vi "Top Level FPGA_w8LED.vi"() -> ()   [LabVIEW 2012]
uses:
  <vilib>/Platform/TimedLoop/XDataNode/timing_clust.ctl
  <vilib>/Platform/TimedLoop/XDataNode/nitl_modes.ctl
  <vilib>/Platform/TimedLoop/XDataNode/wakeup.ctl
  <vilib>/rvi/DataTransferAndStorage/Container/Common/niFpgaContainerMetaDataKey.ctl
  <vilib>/rvi/DataTransferAndStorage/Container/Common/niFpgaContainerState.ctl
  <vilib>/rvi/DataTransferAndStorage/Container/Common/niFpgaDataTypeControl.ctl
  <vilib>/rvi/DataTransferAndStorage/Container/Common/niFpgaContainerImplementationControl.ctl
  <vilib>/rvi/DataTransferAndStorage/Container/Common/niFpgaContainerArbitrationOptionsControl.ctl
  <vilib>/rvi/DataTransferAndStorage/Container/Common/niFpgaTransferTypeControl.ctl
  <vilib>/rvi/DataTransferAndStorage/Container/Common/niFpgaContainerInitializationParameters.ctl
  <vilib>/rvi/Memory/Memory_Types/niFpgaMemoryInterfaceConfiguration.ctl
  <vilib>/rvi/FIFO/Fifo_Types/niFpgaFifoControlLogicControl.ctl
  <vilib>/rvi/eio/common/nirviEmuTemplateMethod_errors.vi
  <vilib>/rvi/FIFO/Fifo_Resource/nirvififoEmulationSetSize.vi
  <vilib>/rvi/DataTransferAndStorage/Container/Common/niFpgaContainerGetUniqueNameForEmu.vi
  <vilib>/rvi/Emulation/niFpgaSctlEmulationRegisterWithScheduler.vi
  <vilib>/rvi/Emulation/niFpgaSctlEmulationScheduler.vi
  <vilib>/rvi/DataTransferAndStorage/Container/Common/niFpgaContainerSetEmuInfo.vi
  <vilib>/rvi/eio/common/nirviEmuReportErrorAndStop.vi
  <vilib>/rvi/Emulation/niFpgaSctlEmulationFifoFullMgr.vi
  <vilib>/rvi/errors/niFpgaSetErrorForExecOnDevCompSimple.vi
  <vilib>/rvi/Memory/Memory_Emulation/niFpgaMemoryEmulationCacheClearOnFirstRun.vi
  <vilib>/rvi/Memory/Memory_Emulation/nirvimemoryEmulationManagerCache_MakeExclusive.vi
  <vilib>/rvi/Memory/Memory_Emulation/niFpgaMemoryEmulationValidateCache.vi
  <vilib>/rvi/Memory/Memory_Emulation/nirvimemoryEmulationManagerCache_ReleaseExclusive.vi
  <vilib>/rvi/Memory/Memory_Emulation/nirvimemoryEmulationManagerCache_InsertValue.vi
  <vilib>/Utility/error.llb/Clear Errors.vi
  <vilib>/rvi/Memory/Memory_Emulation/nirvimemoryEmulationManagerCache_GetValue.vi
  <vilib>/rvi/Emulation/niFpgaSctlEmulationResourceMgr.vi
  <vilib>/eio/EIONode/EIONode.xnode
  <vilib>/Platform/TimedLoop/XDataNode/XDataNode.xnode
  <vilib>/rvi/DataTransferAndStorage/Container/XNode/niFpgaContainer.xnode
  <vilib>/rvi/FIFO/Fifo_Resource/nirvififoEmulationClear.vi
  <vilib>/rvi/LocalResourceManager/LocalResourceManager.xnode
  <vilib>/rvi/FIFO/Fifo_Resource/nirvififoEmulationRead.vi
  <vilib>/rvi/Memory/Memory_Emulation/nirvimemoryEmulation.vi
  <vilib>/rvi/FIFO/Fifo_Resource/nirvififoEmulationWrite.vi
  <vilib>/Platform/TimedLoop/XDataNode/XDNodeRunTimeDep.lvlib
panel:
  out "IO Module\\ADC Error A":bool
  out "IO Module\\ADC Error B":bool
  out "IO Module\\Pll Unlocked":bool
  in  "Record Size only data":u32=95
  out "DMA FIFO Timed Out?":bool
  in  "circular buffer length":u32=1000
  in  "location":i16(ring) items=["Purdue", "NIKHEF", "Zurich", "???"]
  in  "Trigger 0":i16=4000
  in  "Trigger 1":i16=4000
  in  "Trigger 2":i16=4000
  in  "Trigger 3":i16=4000
  in  "Trigger 4":i16=4000
  in  "Trigger 5":i16=4000
  in  "Trigger 6":i16=4000
  in  "Trigger 7":i16=4000
  in  "# of pretrigger":u32=20
  in  "initial value":u64
  in  "channel 0 on/off":bool
  in  "channel 2 on/off":bool
  in  "channel 1 on/off":bool
  in  "channel 3 on/off":bool
  in  "channel 4 on/off":bool
  in  "channel 5 on/off":bool
  in  "channel 6 on/off":bool
  in  "channel 7 on/off":bool
  out "Is Channel 0 Test Pulse?":bool
  in  "Testpulse duration (20 ns ticks)":u32=1
  in  "Testpulse Separation (20 ns ticks)":u32=500
  in  "Testpulse Time Delay (20 ns ticks)":u32=15
  out "Is Channel 1 Test Pulse?":bool
  in  "Testpulser On/Off":bool
  out "Is Channel 2 Test Pulse?":bool
  out "Is Channel 3 Test Pulse?":bool
  out "Is Channel 4 Test Pulse?":bool
  out "Is Channel 5 Test Pulse?":bool
  out "Is Channel 6 Test Pulse?":bool
  out "Is Channel 7 Test Pulse?":bool
  out "Init Done":bool
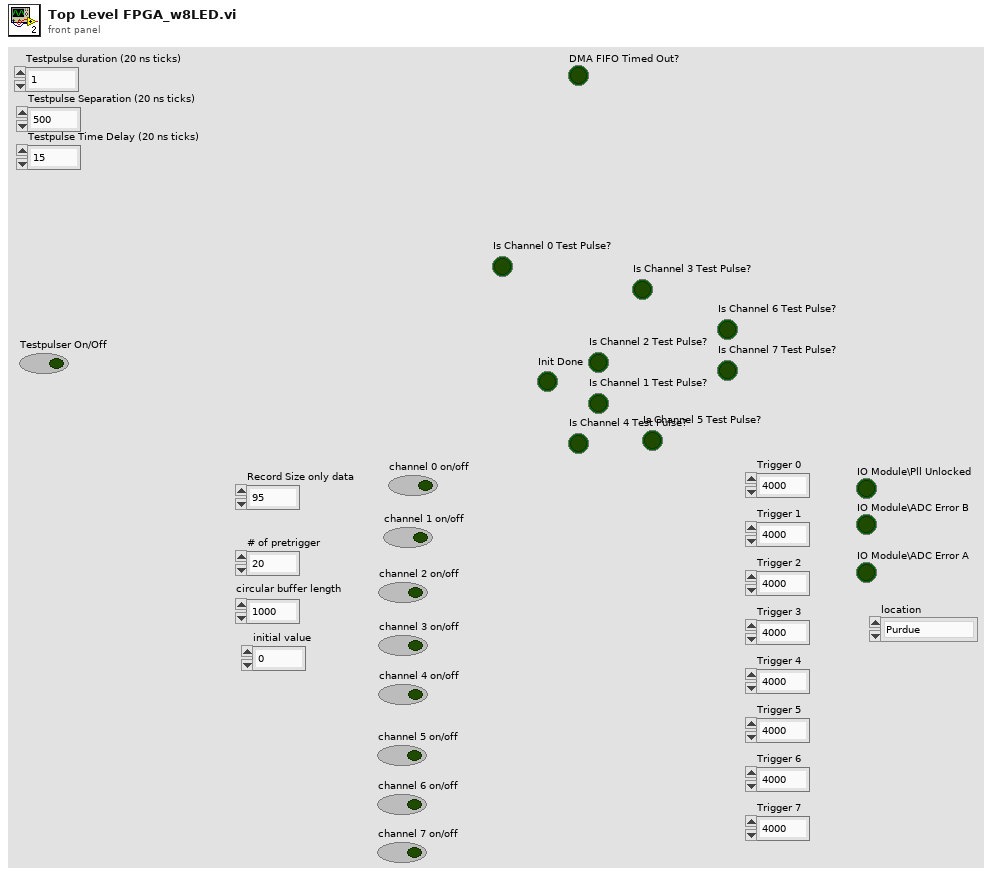
[diagram p1: front panel]
types:
  T1 = typedef "XDNodeRunTimeDep.lvlib/timing_clust.ctl" = cluster{"Expected End [f-1]":u64, "Actual End [f-1]":u64, "Finished Late? [f-1]":bool, "Expected End [i-1]":u64, "Actual End [i-1]":u64, "Finished Late? [i-1]":bool, "Expected Start [i]":u64, "Actual Start [i]":u64, "Expected Start [f]":u64, "Actual Start [f]":u64, "Source Name":string, "Structure Name":string, "Period":i64, "Deadline":i64, "Offset":i64, "Start":i64, "Priority":i32, "Timeout":i32, "Mode":T2, "Wakeup Reason":T3, "Error":errorcluster, "Source Type":string, "Secondary Source Type":string, "Global End Time":u64, "Global Start Time":u64, "Frame Duration":u64, "Iteration Duration":u64, "Assigned CPU":i32, "I/O Scan Engine Mode":u32}
  T2 = typedef "XDNodeRunTimeDep.lvlib/nitl_modes.ctl" = enum32{"No Change", "Process missed periods, maintain original phase", "Discard missed periods, maintain original phase", "Process missed periods, ignore original phase", "Discard missed periods, ignore original phase"}
  T3 = typedef "XDNodeRunTimeDep.lvlib/wakeup.ctl" = enum32{"Normal", "Aborted", "Asynchronous wakeup", "Timing source error", "Timed loop error", "Timeout"}
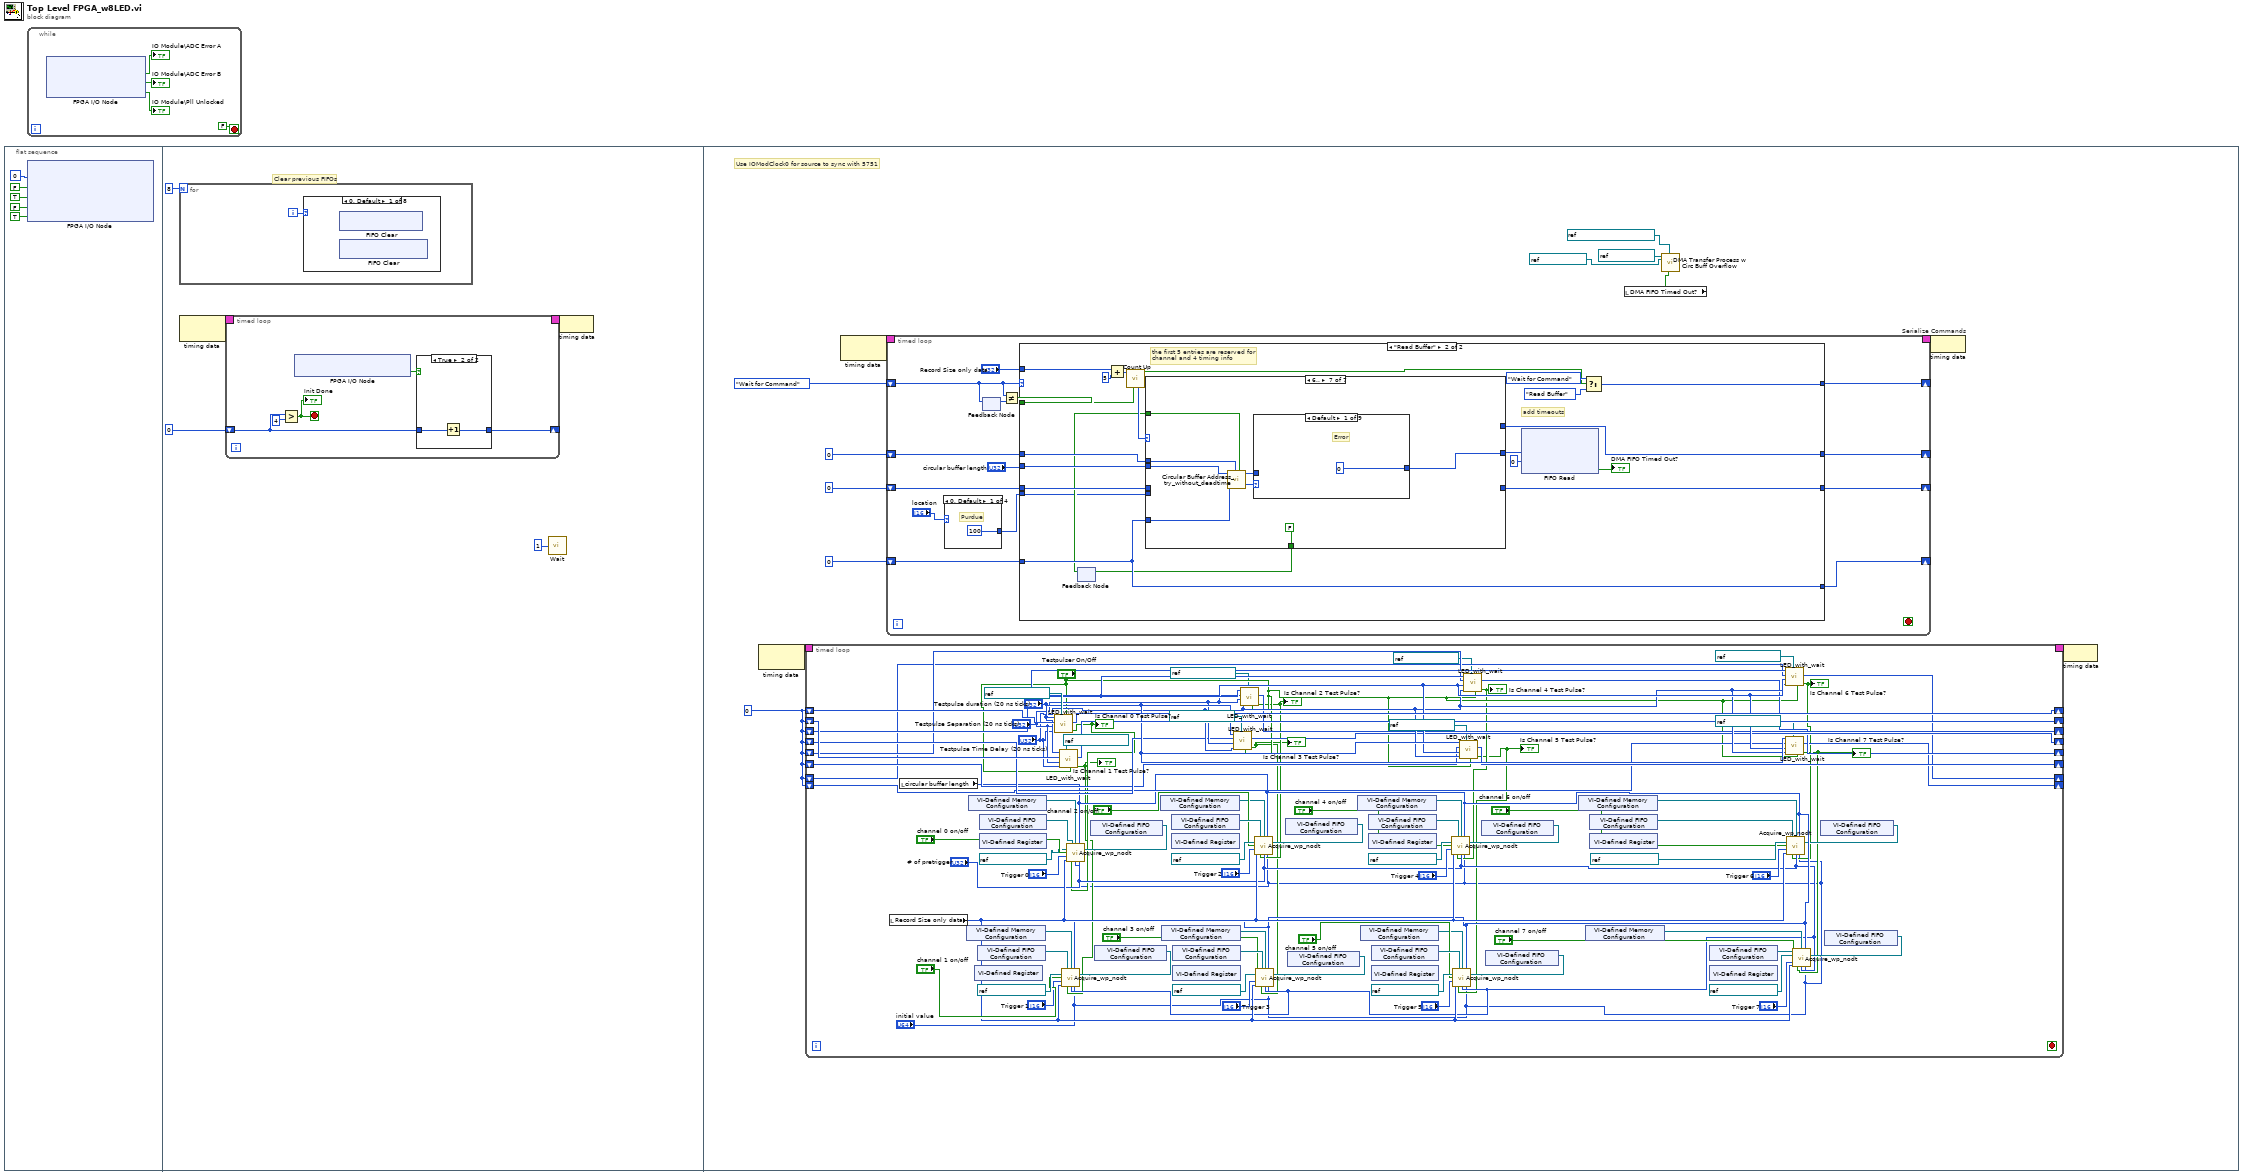
[diagram p0: block diagram]
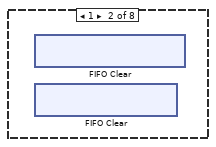
[diagram p2: hidden frame]
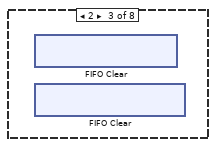
[diagram p3: hidden frame]
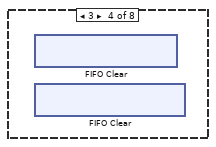
[diagram p4: hidden frame]
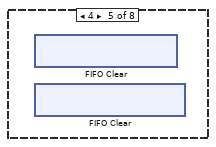
[diagram p5: hidden frame]
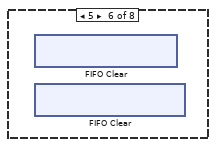
[diagram p6: hidden frame]
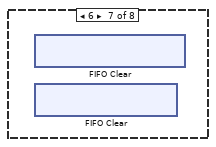
[diagram p7: hidden frame]
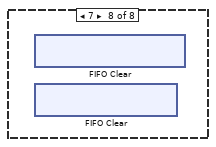
[diagram p8: hidden frame]
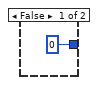
[diagram p9: hidden frame]
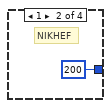
[diagram p10: hidden frame]
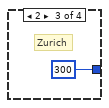
[diagram p11: hidden frame]
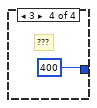
[diagram p12: hidden frame]
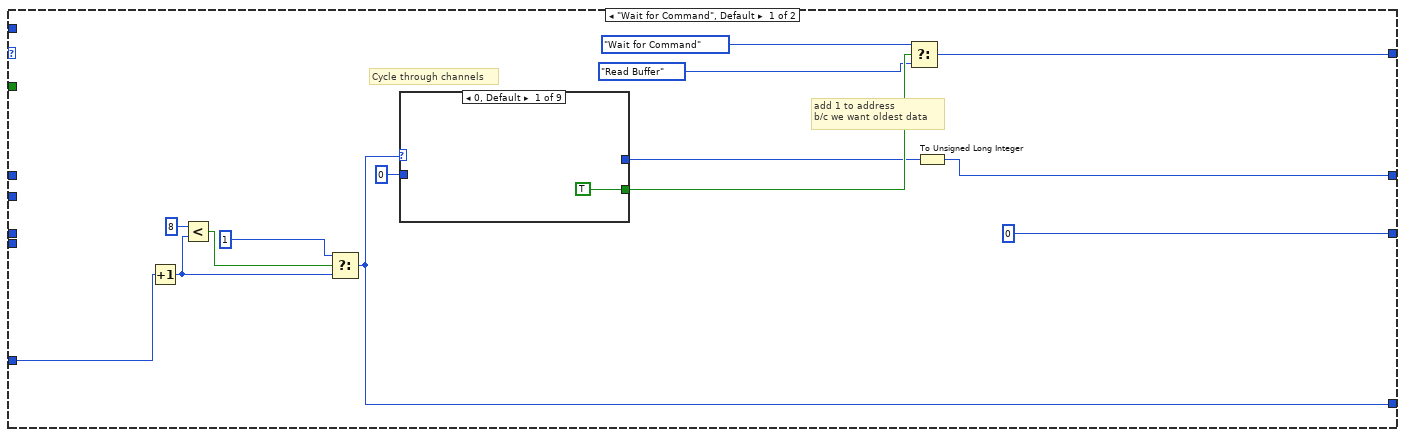
[diagram p13: hidden frame]
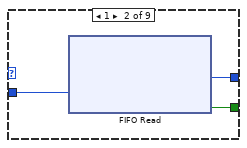
[diagram p14: hidden frame]
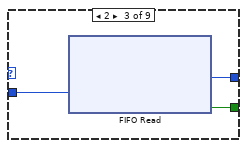
[diagram p15: hidden frame]
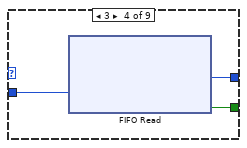
[diagram p16: hidden frame]
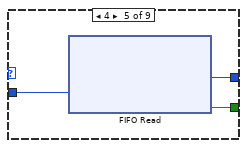
[diagram p17: hidden frame]
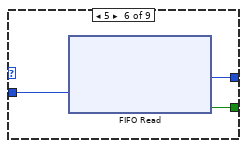
[diagram p18: hidden frame]
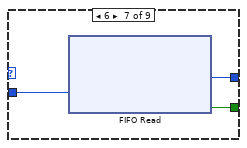
[diagram p19: hidden frame]
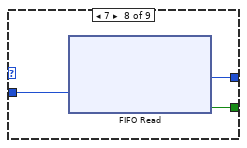
[diagram p20: hidden frame]
diagram:
  n1 = flat-sequence {
    frame #0 {
      n2 = xnode "FPGA I/O Node"("IO Module\\Sample Clock Select"=u8 0 ("IO Module\\Sample Clock Select"), "IO Module\\Force Initialization"=FALSE ("IO Module\\Force Initialization"), "IO Module\\Force Initialization"=TRUE ("IO Module\\Force Initialization"), "IO Module\\Force Initialization"=FALSE ("IO Module\\Force Initialization"), "IO Module\\Digital Output Enable"=TRUE ("IO Module\\Digital Output Enable")) -> ()  [unwired: 5 in, 5 out]
    }
    frame #1 {
      # "Clear previous FIFOs"
      n3 = for {
        N: 8 -> [_]
        i -> [w11]
        n4 = case shown="0, Default" w11 {
          frame 0, Default {
            n5 = xnode ("FIFO Clear")() -> ()  [unwired: 1 in, 1 out]
            n6 = xnode ("FIFO Clear")() -> ()  [unwired: 1 in, 1 out]
          }
          frame 1 {
            n7 = xnode ("FIFO Clear")() -> ()  [unwired: 1 in, 1 out]
            n8 = xnode ("FIFO Clear")() -> ()  [unwired: 1 in, 1 out]
          }
          frame 2 {
            n9 = xnode ("FIFO Clear")() -> ()  [unwired: 1 in, 1 out]
            n10 = xnode ("FIFO Clear")() -> ()  [unwired: 1 in, 1 out]
          }
          frame 3 {
            n11 = xnode ("FIFO Clear")() -> ()  [unwired: 1 in, 1 out]
            n12 = xnode ("FIFO Clear")() -> ()  [unwired: 1 in, 1 out]
          }
          frame 4 {
            n13 = xnode ("FIFO Clear")() -> ()  [unwired: 1 in, 1 out]
            n14 = xnode ("FIFO Clear")() -> ()  [unwired: 1 in, 1 out]
          }
          frame 5 {
            n15 = xnode ("FIFO Clear")() -> ()  [unwired: 1 in, 1 out]
            n16 = xnode ("FIFO Clear")() -> ()  [unwired: 1 in, 1 out]
          }
          frame 6 {
            n17 = xnode ("FIFO Clear")() -> ()  [unwired: 1 in, 1 out]
            n18 = xnode ("FIFO Clear")() -> ()  [unwired: 1 in, 1 out]
          }
          frame 7 {
            n19 = xnode ("FIFO Clear")() -> ()  [unwired: 1 in, 1 out]
            n20 = xnode ("FIFO Clear")() -> ()  [unwired: 1 in, 1 out]
          }
        }
      }
      n21 = node-c288() -> (w10:T1)  [unwired: 1 in]
      n22 = timed-loop {
        shift-right: [w15] -> _
        shift-left: u16 0 -> [w14]
        timing: w10 -> [_]
        timing-out: [_] -> w9
        stop <- w12 stop-if-true
        n23 = Greater?(x=w14, y=u16 4) -> (0:w12:bool)
        "Init Done" <- w12
        n24 = xnode "FPGA I/O Node"() -> ("IO Module\\Initialization Done"=w16:bool)  [unwired: 1 in, 1 out]
        n25 = case shown="True" w16 {
          tunnel: [u16 0 w19] -> w15
          tunnel: w14 -> [_ w18]
          frame False {
          }
          frame True {
            n26 = Increment(x=w18) -> (x+1=w19:u16)
          }
        }
      }
      n27 = call "Wait"("Count(mSec)"=u32 1) -> ()  [unwired: 1 out]
      n28 = node-c288(w9) -> ()
    }
    frame #2 {
      w24 = u64 0 ("Total number of pulses sent")
      # "Use IOModClock0 for source to sync with 5751"
      n29 = node-c288() -> (w30:T1)  [unwired: 1 in]
      n30 = timed-loop {
        timing: w30 -> [_]
        timing-out: [_] -> w29
        shift-right: [w98] -> _
        shift-left: w24 -> [w99]
        shift-right: [w94] -> _
        shift-left: w24 -> [w95]
        shift-right: [w89] -> _
        shift-left: w24 -> [w90]
        shift-right: [w88] -> _
        shift-left: w24 -> [w83]
        shift-right: [w87] -> _
        shift-left: w24 -> [w82]
        shift-right: [w86] -> _
        shift-left: w24 -> [w81]
        shift-right: [w85] -> _
        shift-left: w24 -> [w80]
        shift-right: [w84] -> _
        shift-left: w24 -> [w79]
        stop <- _ stop-if-true
        n31 = local read "Record Size only data"() -> (w100:u32)
        n32 = local read "circular buffer length"() -> (w55:u32)
        n33 = xnode "VI-Defined Memory Configuration"() -> ("Memory Out"=w56:refnum<k21>)
        n34 = xnode "VI-Defined Memory Configuration"() -> ("Memory Out"=w63:refnum<k21>)
        n35 = xnode "VI-Defined Register"() -> ()  [unwired: 1 out]
        n36 = xnode "VI-Defined FIFO Configuration"() -> ("FIFO Out"=w124:refnum<k21>)
        n37 = xnode "VI-Defined FIFO Configuration"() -> ("FIFO Out"=w101:refnum<k21>)
        n38 = xnode "VI-Defined Register"() -> ()  [unwired: 1 out]
        n39 = call "LED_with_wait.vi"("Testpulser On/Off"="Testpulser On/Off", "FPGA I/O In"=refnum<k21> "IO Module\\D0 0", "Testpulse Time Delay (20 ns ticks)"="Testpulse Time Delay (20 ns ticks)", "Testpulse Separation (20 ns ticks)"="Testpulse Separation (20 ns ticks)", "Total number of pulses input"=w99, "Testpulse duration (20 ns ticks)"="Testpulse duration (20 ns ticks)") -> ("Is Test Pulse?"=w45:bool, "Total number of pulses sent"=w98:u64)  [unwired: 4 in]
        "Is Channel 0 Test Pulse?" <- w45
        n40 = call "LED_with_wait.vi"("Testpulser On/Off"="Testpulser On/Off", "FPGA I/O In"=refnum<k21> "IO Module\\D0 1", "Testpulse Time Delay (20 ns ticks)"="Testpulse Time Delay (20 ns ticks)", "Testpulse Separation (20 ns ticks)"="Testpulse Separation (20 ns ticks)", "Total number of pulses input"=w95, "Testpulse duration (20 ns ticks)"="Testpulse duration (20 ns ticks)") -> ("Is Test Pulse?"=w44:bool, "Total number of pulses sent"=w94:u64)  [unwired: 4 in]
        "Is Channel 1 Test Pulse?" <- w44
        n41 = xnode "VI-Defined FIFO Configuration"() -> ("FIFO Out"=w53:refnum<k21>)
        n42 = call "Acquire_wp_nodt.vi"("Command FIFO"=w101, "Circular Buffer Mem"=w63, "circular buffer length"=w55, "FPGA I/O In"=refnum<k21> "IO Module\\AI A0", "Timing FIFO"=w53, "channel on/off"="channel 0 on/off", "Trigger"="Trigger 0", "Samples to Acquire"=w100, "Is Test Pulse?"=w45, "# of pretrigger"="# of pretrigger", "timing"="initial value") -> ()  [unwired: 5 in]
        n43 = xnode "VI-Defined FIFO Configuration"() -> ("FIFO Out"=w54:refnum<k21>)
        n44 = call "Acquire_wp_nodt.vi"("Command FIFO"=w124, "Circular Buffer Mem"=w56, "circular buffer length"=w55, "FPGA I/O In"=refnum<k21> "IO Module\\AI A1", "Timing FIFO"=w54, "channel on/off"="channel 1 on/off", "Trigger"="Trigger 1", "Samples to Acquire"=w100, "Is Test Pulse?"=w44, "# of pretrigger"="# of pretrigger", "timing"="initial value") -> ()  [unwired: 5 in]
        n45 = xnode "VI-Defined Memory Configuration"() -> ("Memory Out"=w62:refnum<k21>)
        n46 = xnode "VI-Defined Memory Configuration"() -> ("Memory Out"=w57:refnum<k21>)
        n47 = xnode "VI-Defined FIFO Configuration"() -> ("FIFO Out"=w122:refnum<k21>)
        n48 = xnode "VI-Defined Register"() -> ()  [unwired: 1 out]
        n49 = xnode "VI-Defined FIFO Configuration"() -> ("FIFO Out"=w123:refnum<k21>)
        n50 = xnode "VI-Defined Register"() -> ()  [unwired: 1 out]
        n51 = call "LED_with_wait.vi"("Testpulser On/Off"="Testpulser On/Off", "FPGA I/O In"=refnum<k21> "IO Module\\D0 3", "Testpulse Time Delay (20 ns ticks)"="Testpulse Time Delay (20 ns ticks)", "Testpulse Separation (20 ns ticks)"="Testpulse Separation (20 ns ticks)", "Total number of pulses input"=w83, "Testpulse duration (20 ns ticks)"="Testpulse duration (20 ns ticks)") -> ("Is Test Pulse?"=w42:bool, "Total number of pulses sent"=w88:u64)  [unwired: 4 in]
        "Is Channel 3 Test Pulse?" <- w42
        n52 = call "LED_with_wait.vi"("Testpulser On/Off"="Testpulser On/Off", "FPGA I/O In"=refnum<k21> "IO Module\\D0 2", "Testpulse Time Delay (20 ns ticks)"="Testpulse Time Delay (20 ns ticks)", "Testpulse Separation (20 ns ticks)"="Testpulse Separation (20 ns ticks)", "Total number of pulses input"=w90, "Testpulse duration (20 ns ticks)"="Testpulse duration (20 ns ticks)") -> ("Is Test Pulse?"=w43:bool, "Total number of pulses sent"=w89:u64)  [unwired: 4 in]
        "Is Channel 2 Test Pulse?" <- w43
        n53 = xnode "VI-Defined FIFO Configuration"() -> ("FIFO Out"=w52:refnum<k21>)
        n54 = call "Acquire_wp_nodt.vi"("Command FIFO"=w122, "Circular Buffer Mem"=w62, "circular buffer length"=w55, "FPGA I/O In"=refnum<k21> "IO Module\\AI A2", "Timing FIFO"=w52, "channel on/off"="channel 2 on/off", "Trigger"="Trigger 2", "Samples to Acquire"=w100, "Is Test Pulse?"=w43, "# of pretrigger"="# of pretrigger", "timing"="initial value") -> ()  [unwired: 5 in]
        n55 = xnode "VI-Defined FIFO Configuration"() -> ("FIFO Out"=w51:refnum<k21>)
        n56 = call "Acquire_wp_nodt.vi"("Command FIFO"=w123, "Circular Buffer Mem"=w57, "circular buffer length"=w55, "FPGA I/O In"=refnum<k21> "IO Module\\AI A3", "Timing FIFO"=w51, "channel on/off"="channel 3 on/off", "Trigger"="Trigger 3", "Samples to Acquire"=w100, "Is Test Pulse?"=w42, "# of pretrigger"="# of pretrigger", "timing"="initial value") -> ()  [unwired: 5 in]
        n57 = xnode "VI-Defined Memory Configuration"() -> ("Memory Out"=w61:refnum<k21>)
        n58 = xnode "VI-Defined Memory Configuration"() -> ("Memory Out"=w58:refnum<k21>)
        n59 = xnode "VI-Defined Register"() -> ()  [unwired: 1 out]
        n60 = xnode "VI-Defined FIFO Configuration"() -> ("FIFO Out"=w118:refnum<k21>)
        n61 = xnode "VI-Defined FIFO Configuration"() -> ("FIFO Out"=w119:refnum<k21>)
        n62 = xnode "VI-Defined Register"() -> ()  [unwired: 1 out]
        n63 = call "LED_with_wait.vi"("Testpulser On/Off"="Testpulser On/Off", "FPGA I/O In"=refnum<k21> "IO Module\\D0 5", "Testpulse Time Delay (20 ns ticks)"="Testpulse Time Delay (20 ns ticks)", "Testpulse Separation (20 ns ticks)"="Testpulse Separation (20 ns ticks)", "Total number of pulses input"=w81, "Testpulse duration (20 ns ticks)"="Testpulse duration (20 ns ticks)") -> ("Is Test Pulse?"=w40:bool, "Total number of pulses sent"=w86:u64)  [unwired: 4 in]
        "Is Channel 5 Test Pulse?" <- w40
        n64 = call "LED_with_wait.vi"("Testpulser On/Off"="Testpulser On/Off", "FPGA I/O In"=refnum<k21> "IO Module\\D0 4", "Testpulse Time Delay (20 ns ticks)"="Testpulse Time Delay (20 ns ticks)", "Testpulse Separation (20 ns ticks)"="Testpulse Separation (20 ns ticks)", "Total number of pulses input"=w82, "Testpulse duration (20 ns ticks)"="Testpulse duration (20 ns ticks)") -> ("Is Test Pulse?"=w41:bool, "Total number of pulses sent"=w87:u64)  [unwired: 4 in]
        "Is Channel 4 Test Pulse?" <- w41
        n65 = xnode "VI-Defined FIFO Configuration"() -> ("FIFO Out"=w47:refnum<k21>)
        n66 = call "Acquire_wp_nodt.vi"("Command FIFO"=w118, "Circular Buffer Mem"=w61, "circular buffer length"=w55, "FPGA I/O In"=refnum<k21> "IO Module\\AI A4", "Timing FIFO"=w47, "channel on/off"="channel 4 on/off", "Trigger"="Trigger 4", "Samples to Acquire"=w100, "Is Test Pulse?"=w41, "# of pretrigger"="# of pretrigger", "timing"="initial value") -> ()  [unwired: 5 in]
        n67 = xnode "VI-Defined FIFO Configuration"() -> ("FIFO Out"=w50:refnum<k21>)
        n68 = call "Acquire_wp_nodt.vi"("Command FIFO"=w119, "Circular Buffer Mem"=w58, "circular buffer length"=w55, "FPGA I/O In"=refnum<k21> "IO Module\\AI A5", "Timing FIFO"=w50, "channel on/off"="channel 5 on/off", "Trigger"="Trigger 5", "Samples to Acquire"=w100, "Is Test Pulse?"=w40, "# of pretrigger"="# of pretrigger", "timing"="initial value") -> ()  [unwired: 5 in]
        n69 = xnode "VI-Defined Memory Configuration"() -> ("Memory Out"=w60:refnum<k21>)
        n70 = xnode "VI-Defined Memory Configuration"() -> ("Memory Out"=w59:refnum<k21>)
        n71 = xnode "VI-Defined FIFO Configuration"() -> ("FIFO Out"=w121:refnum<k21>)
        n72 = xnode "VI-Defined Register"() -> ()  [unwired: 1 out]
        n73 = xnode "VI-Defined FIFO Configuration"() -> ("FIFO Out"=w120:refnum<k21>)
        n74 = xnode "VI-Defined Register"() -> ()  [unwired: 1 out]
        n75 = call "LED_with_wait.vi"("Testpulser On/Off"="Testpulser On/Off", "FPGA I/O In"=refnum<k21> "IO Module\\D0 6", "Testpulse Time Delay (20 ns ticks)"="Testpulse Time Delay (20 ns ticks)", "Testpulse Separation (20 ns ticks)"="Testpulse Separation (20 ns ticks)", "Total number of pulses input"=w80, "Testpulse duration (20 ns ticks)"="Testpulse duration (20 ns ticks)") -> ("Is Test Pulse?"=w39:bool, "Total number of pulses sent"=w85:u64)  [unwired: 4 in]
        "Is Channel 6 Test Pulse?" <- w39
        n76 = call "LED_with_wait.vi"("Testpulser On/Off"="Testpulser On/Off", "FPGA I/O In"=refnum<k21> "IO Module\\D0 7", "Testpulse Time Delay (20 ns ticks)"="Testpulse Time Delay (20 ns ticks)", "Testpulse Separation (20 ns ticks)"="Testpulse Separation (20 ns ticks)", "Total number of pulses input"=w79, "Testpulse duration (20 ns ticks)"="Testpulse duration (20 ns ticks)") -> ("Is Test Pulse?"=w38:bool, "Total number of pulses sent"=w84:u64)  [unwired: 4 in]
        "Is Channel 7 Test Pulse?" <- w38
        n77 = xnode "VI-Defined FIFO Configuration"() -> ("FIFO Out"=w48:refnum<k21>)
        n78 = call "Acquire_wp_nodt.vi"("Command FIFO"=w121, "Circular Buffer Mem"=w60, "circular buffer length"=w55, "FPGA I/O In"=refnum<k21> "IO Module\\AI A6", "Timing FIFO"=w48, "channel on/off"="channel 6 on/off", "Trigger"="Trigger 6", "Samples to Acquire"=w100, "Is Test Pulse?"=w39, "# of pretrigger"="# of pretrigger", "timing"="initial value") -> ()  [unwired: 5 in]
        n79 = xnode "VI-Defined FIFO Configuration"() -> ("FIFO Out"=w49:refnum<k21>)
        n80 = call "Acquire_wp_nodt.vi"("Command FIFO"=w120, "Circular Buffer Mem"=w59, "circular buffer length"=w55, "FPGA I/O In"=refnum<k21> "IO Module\\AI A7", "Timing FIFO"=w49, "channel on/off"="channel 7 on/off", "Trigger"="Trigger 7", "Samples to Acquire"=w100, "Is Test Pulse?"=w38, "# of pretrigger"="# of pretrigger", "timing"="initial value") -> ()  [unwired: 5 in]
      }
      n81 = node-c288() -> (w32:T1)  [unwired: 1 in]
      n82 = timed-loop "Serialize Commands" {
        timing: w32 -> [_]
        timing-out: [_] -> w31
        shift-right: [w905] -> _
        shift-left: enum16{"Wait for Command", "Read Buffer"}."Wait for Command" -> [w903]
        shift-right: [w909] -> _
        shift-left: u32 0 ("Element") -> [w908]
        shift-right: [w907] -> _
        shift-left: u8 0 ("t") -> [w906]
        shift-right: [w900] -> _
        shift-left: u64 0 ("Element") -> [w899]
        stop <- _ stop-if-true
        n83 = case shown="0, Default" "location" {
          tunnel: [i16 100 i16 200 i16 300 i16 400] -> w897
          frame 0, Default {
            # "Purdue"
          }
          frame 1 {
            # "NIKHEF"
          }
          frame 2 {
            # "Zurich"
          }
          frame 3 {
            # "???"
          }
        }
        n84 = feedback-in #1(w903) -> ()
        n85 = feedback #1() -> (w904:enum16{"Wait for Command", "Read Buffer"})  [unwired: 1 in]
        n86 = Not Equal?(x=w903, y=w904) -> (x != y?=w901:bool)
        n87 = case shown="\"Read Buffer\"" w903 {
          tunnel: "Record Size only data" -> [_ w963]
          tunnel: [w917 w973] -> w907
          tunnel: w906 -> [w919 w973]
          tunnel: [w920 w958] -> w909
          tunnel: w908 -> [_ w972]
          tunnel: [w923 w974] -> w905
          tunnel: "circular buffer length" -> [_ w971]
          tunnel: w901 -> [_ w965]
          tunnel: [u64 0 ("Element") w960] -> w900
          tunnel: w899 -> [_ w959]
          tunnel: w897 -> [_ w954]
          frame "Wait for Command", Default {
            # "add 1 to address\nb/c we want oldest data"
            # "Cycle through channels"
            n88 = Increment(x=w919) -> (x+1=w918:u8)
            n89 = Less?(x=u8 8, y=w918) -> (x < y?=w927:bool)
            n90 = Select(t=u8 1, s=w927, f=w918) -> (s? t:f=w917:u8)
            n91 = case shown="0, Default" w917 {
              tunnel: [TRUE ("Timed Out?") w932 w933 w936 w939 w942 w945 w948 w951] -> w924
              tunnel: 0 ("Timeout") -> [_ w931 w935 w938 w941 w944 w947 w950 w953]
              tunnel: [_ w930 w934 w937 w940 w943 w946 w949 w952] -> w916
              frame 0, Default {
              }
              frame 1 {
                n92 = xnode ("FIFO Read")("Timeout"=w931) -> ("Element"=w930:i16, "Timed Out?"=w932:bool)  [unwired: 1 in, 1 out]
              }
              frame 2 {
                n93 = xnode ("FIFO Read")("Timeout"=w935) -> ("Element"=w934:i16, "Timed Out?"=w933:bool)  [unwired: 1 in, 1 out]
              }
              frame 3 {
                n94 = xnode ("FIFO Read")("Timeout"=w938) -> ("Element"=w937:i16, "Timed Out?"=w936:bool)  [unwired: 1 in, 1 out]
              }
              frame 4 {
                n95 = xnode ("FIFO Read")("Timeout"=w941) -> ("Element"=w940:i16, "Timed Out?"=w939:bool)  [unwired: 1 in, 1 out]
              }
              frame 5 {
                n96 = xnode ("FIFO Read")("Timeout"=w944) -> ("Element"=w943:i16, "Timed Out?"=w942:bool)  [unwired: 1 in, 1 out]
              }
              frame 6 {
                n97 = xnode ("FIFO Read")("Timeout"=w947) -> ("Element"=w946:i16, "Timed Out?"=w945:bool)  [unwired: 1 in, 1 out]
              }
              frame 7 {
                n98 = xnode ("FIFO Read")("Timeout"=w950) -> ("Element"=w949:i16, "Timed Out?"=w948:bool)  [unwired: 1 in, 1 out]
              }
              frame 8 {
                n99 = xnode ("FIFO Read")("Timeout"=w953) -> ("Element"=w952:i16, "Timed Out?"=w951:bool)  [unwired: 1 in, 1 out]
              }
            }
            n100 = Select(t=enum16{"Wait for Command", "Read Buffer"}."Wait for Command", s=w924, f=enum16{"Wait for Command", "Read Buffer"}."Read Buffer") -> (s? t:f=w923:enum16{"Wait for Command", "Read Buffer"})
            n101 = To Unsigned Long Integer(number=w916) -> (unsigned 32bit integer=w920:u32)
          }
          frame "Read Buffer" {
            # "the first 5 entries are reserved for channel and 4 timing info"
            # "add timeouts"
            n102 = feedback #2() -> (w957:bool)  [unwired: 1 in]
            n103 = Add(x=w963, y=u32 5) -> (x+y=w961:u32)
            n104 = call "Count Up.vi"("Reset?"=w965, "goal"=w961) -> ("Count Met"=w967:bool, "count"=w964:u32)  [unwired: 8 in]
            n105 = case shown="6.." w964 {
              tunnel: w973 -> [_ w983 w990 _ _ _ w1029]
              tunnel: w972 -> [_ w987 w992 w1013 w1019 w1025 w1035]
              tunnel: w971 -> [_ _ _ _ _ _ w1034]
              tunnel: [i16 0 ("Data") w984 w994 w1011 w1017 w1023 w1030] -> w966
              tunnel: w957 -> [_ _ _ _ _ _ w1032]
              tunnel: [u64 0 ("Element") _ w991 w1014 w1020 w1026 _] -> w960
              tunnel: w959 -> [_ _ _ w1014 w1020 w1026 _]
              tunnel: [u32 0 ("Element") w987 w992 w1013 w1019 w1025 _] -> w958
              tunnel: [FALSE FALSE FALSE FALSE FALSE TRUE FALSE] -> w956
              tunnel: w954 -> [_ w979 _ _ _ _ _]
              frame 0, Default {
              }
              frame 1 {
                w985 = u16 0 items=["Header Information", "Particle Pulse", "Test Pulse"] ("Pulse Type")
                n106 = Decrement(x=w983) -> (x-1=w982:u8)
                n107 = To Word Integer(number=w982) -> (16bit integer=w981:i16)
                n108 = Add(x=w979, y=w981) -> (x+y=w980:i16)
                n109 = call "bitmanip.vi"("Pulse Type"=w985, "Integer to be written"=w980) -> ("Integer Written"=w984:i16)  [unwired: 2 in]
              }
              frame 2 {
                # "reads out the lsb of the timing information"
                n110 = case shown="1" w990 {
                  tunnel: [_ w995 w997 w999 w1001 w1003 w1005 w1007 w1009] -> w991
                  frame Default {
                  }
                  frame 1 {
                    n111 = xnode ("FIFO Read")("Timeout"=0) -> ("Element"=w995:u64)  [unwired: 1 in, 2 out]
                  }
                  frame 2 {
                    n112 = xnode ("FIFO Read")("Timeout"=0) -> ("Element"=w997:u64)  [unwired: 1 in, 2 out]
                  }
                  frame 3 {
                    n113 = xnode ("FIFO Read")("Timeout"=0) -> ("Element"=w999:u64)  [unwired: 1 in, 2 out]
                  }
                  frame 4 {
                    n114 = xnode ("FIFO Read")("Timeout"=0) -> ("Element"=w1001:u64)  [unwired: 1 in, 2 out]
                  }
                  frame 5 {
                    n115 = xnode ("FIFO Read")("Timeout"=0) -> ("Element"=w1003:u64)  [unwired: 1 in, 2 out]
                  }
                  frame 6 {
                    n116 = xnode ("FIFO Read")("Timeout"=0) -> ("Element"=w1005:u64)  [unwired: 1 in, 2 out]
                  }
                  frame 7 {
                    n117 = xnode ("FIFO Read")("Timeout"=0) -> ("Element"=w1007:u64)  [unwired: 1 in, 2 out]
                  }
                  frame 8 {
                    n118 = xnode ("FIFO Read")("Timeout"=0) -> ("Element"=w1009:u64)  [unwired: 1 in, 2 out]
                  }
                }
                n119 = Split Number(x=w991) -> (hi(x)=w989:u32)  [unwired: 1 out]
                n120 = Split Number(x=w989) -> (hi(x)=w988:u16)  [unwired: 1 out]
                n121 = To Word Integer(number=w988) -> (16bit integer=w994:i16)
              }
              frame 3 {
                n122 = Split Number(x=w1014) -> (hi(x)=w1016:u32)  [unwired: 1 out]
                n123 = Split Number(x=w1016) -> (lo(x)=w1015:u16)  [unwired: 1 out]
                n124 = To Word Integer(number=w1015) -> (16bit integer=w1011:i16)
              }
              frame 4 {
                n125 = Split Number(x=w1020) -> (lo(x)=w1022:u32)  [unwired: 1 out]
                n126 = Split Number(x=w1022) -> (hi(x)=w1021:u16)  [unwired: 1 out]
                n127 = To Word Integer(number=w1021) -> (16bit integer=w1017:i16)
              }
              frame 5 {
                n128 = Split Number(x=w1026) -> (lo(x)=w1028:u32)  [unwired: 1 out]
                n129 = Split Number(x=w1028) -> (lo(x)=w1027:u16)  [unwired: 1 out]
                n130 = To Word Integer(number=w1027) -> (16bit integer=w1023:i16)
              }
              frame 6.. {
                n131 = call "Circular Buffer Address_try_without_deadtime.vi"("Reset?"=w1032, "Starting Address"=w1035, "circular buffer length"=w1034) -> ("Address"=w1033:u32)  [unwired: 8 in]
                n132 = case shown="Default" w1029 {
                  tunnel: w1033 -> [_ w1038 w1040 w1042 w1044 w1046 w1048 w1050 w1052]
                  tunnel: [i16 0 w1037 w1039 w1041 w1043 w1045 w1047 w1049 w1051] -> w1030
                  frame Default {
                    # "Error"
                  }
                  frame 1 {
                    n133 = xnode ("Memory Read")("Address"=w1038) -> ("Data"=w1037:i16)  [unwired: 1 in, 1 out]
                  }
                  frame 2 {
                    n134 = xnode ("Memory Read")("Address"=w1040) -> ("Data"=w1039:i16)  [unwired: 1 in, 1 out]
                  }
                  frame 3 {
                    n135 = xnode ("Memory Read")("Address"=w1042) -> ("Data"=w1041:i16)  [unwired: 1 in, 1 out]
                  }
                  frame 4 {
                    n136 = xnode ("Memory Read")("Address"=w1044) -> ("Data"=w1043:i16)  [unwired: 1 in, 1 out]
                  }
                  frame 5 {
                    n137 = xnode ("Memory Read")("Address"=w1046) -> ("Data"=w1045:i16)  [unwired: 1 in, 1 out]
                  }
                  frame 6 {
                    n138 = xnode ("Memory Read")("Address"=w1048) -> ("Data"=w1047:i16)  [unwired: 1 in, 1 out]
                  }
                  frame 7 {
                    n139 = xnode ("Memory Read")("Address"=w1050) -> ("Data"=w1049:i16)  [unwired: 1 in, 1 out]
                  }
                  frame 8 {
                    n140 = xnode ("Memory Read")("Address"=w1052) -> ("Data"=w1051:i16)  [unwired: 1 in, 1 out]
                  }
                }
              }
            }
            n141 = feedback-in #2(w956) -> ()
            n142 = xnode ("FIFO Read")("Element"=w966, "Timeout"=0) -> ("Timed Out?"=→"DMA FIFO Timed Out?":bool)  [unwired: 1 in, 1 out]
            n143 = Select(t=enum16{"Wait for Command", "Read Buffer"}."Wait for Command", s=w967, f=enum16{"Wait for Command", "Read Buffer"}."Read Buffer") -> (s? t:f=w974:enum16{"Wait for Command", "Read Buffer"})
          }
        }
      }
      n144 = local read "DMA FIFO Timed Out?"() -> (w33:bool)
      n145 = call "DMA Transfer Process w Circ Buff Overflow.vi"("DMA Write Timed Out?"=w33, "Clock Domain"=refnum<k21> "40 MHz Onboard Clock", "Local"=refnum<k21> "To DMA FIFO", "DMA"=refnum<k21> "To Host FIFO") -> ()  [unwired: 8 in]
      n146 = node-c288(w31) -> ()
      n147 = node-c288(w29) -> ()
    }
  }
  n148 = while {
    stop <- FALSE stop-if-true
    n149 = xnode "FPGA I/O Node"() -> ("IO Module\\ADC Error A"=→"IO Module\\ADC Error A":bool, "IO Module\\ADC Error B"=→"IO Module\\ADC Error B":bool, "IO Module\\Pll Unlocked"=→"IO Module\\Pll Unlocked":bool)  [unwired: 3 in, 3 out]
  }
